vi "Next floor logic. 2vi.vi"(9 "Elevator states array":T1[](array[typedef]), 11 "Floors to serve":cluster{"H call":dbl, "Up":bool}[](array[cluster])) -> (1 "Elevator states array out":T1[](array[typedef]), 3 "Floors to serve out":cluster{"H call":dbl, "Up":bool}[](array[cluster]))   [LabVIEW 2019]
uses:
  Type defs/Elevator states.ctl
  Type defs/Elevator position.ctl
  Type defs/Car buttons.ctl
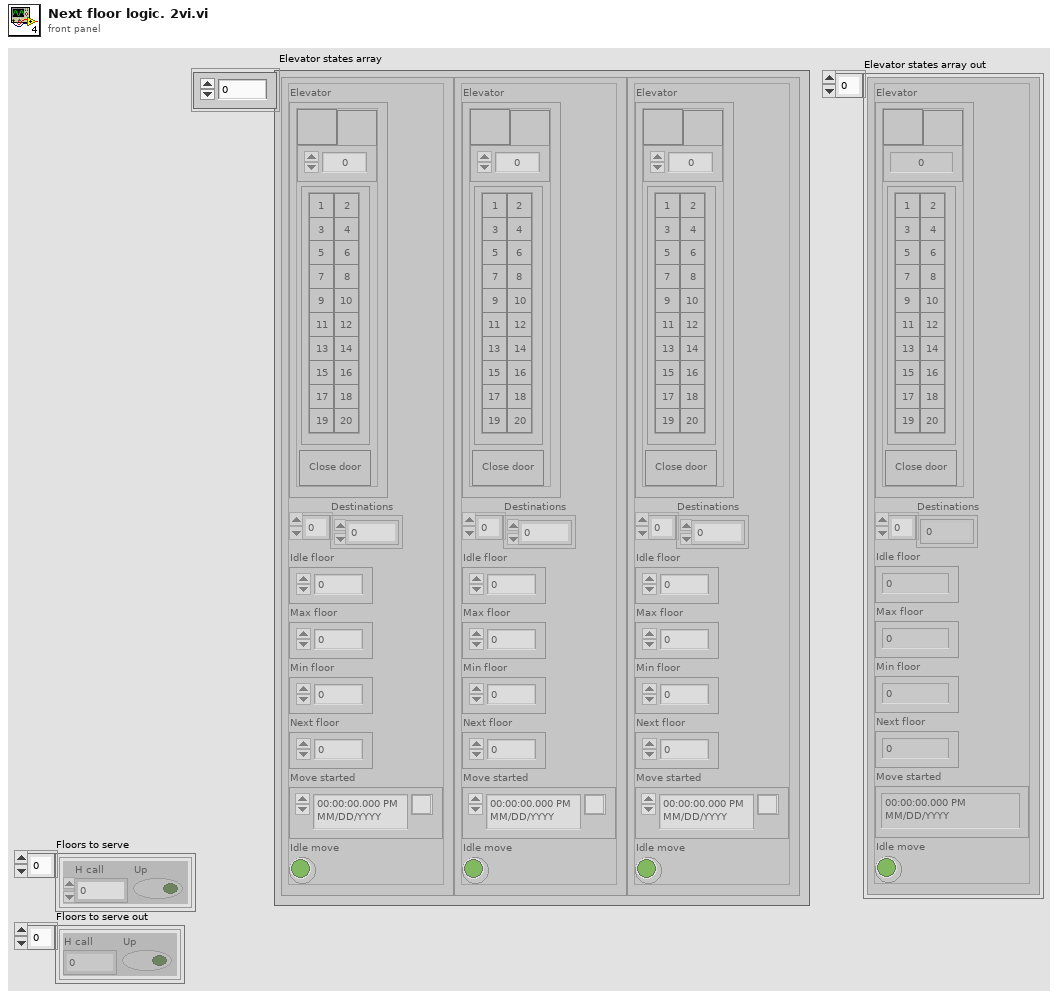
[diagram p1: front panel]
types:
  T1 = typedef "Elevator states.ctl" = cluster{"Elevator":T2, "Destinations":i32[], "Idle floor":u16, "Max floor":u16, "Min floor":u16, "Next floor":u16, "Move started":timestamp, "Idle move":bool}
  T2 = typedef "Elevator position.ctl" = cluster{"Up Button":bool, "Current floor":u16, "Down Button":bool, "Car":T3, "Close door":bool}
  T3 = typedef "Car buttons.ctl" = cluster{"Blank Button":bool, "Blank Button 2":bool, "Blank Button 3":bool, "Blank Button 4":bool, "Blank Button 5":bool, "Blank Button 6":bool, "Blank Button 7":bool, "Blank Button 8":bool, "Blank Button 9":bool, "Blank Button 10":bool, "Blank Button 11":bool, "Blank Button 12":bool, "Blank Button 13":bool, "Blank Button 14":bool, "Blank Button 15":bool, "Blank Button 16":bool, "Blank Button 17":bool, "Blank Button 18":bool, "Blank Button 19":bool, "Blank Button 20":bool}
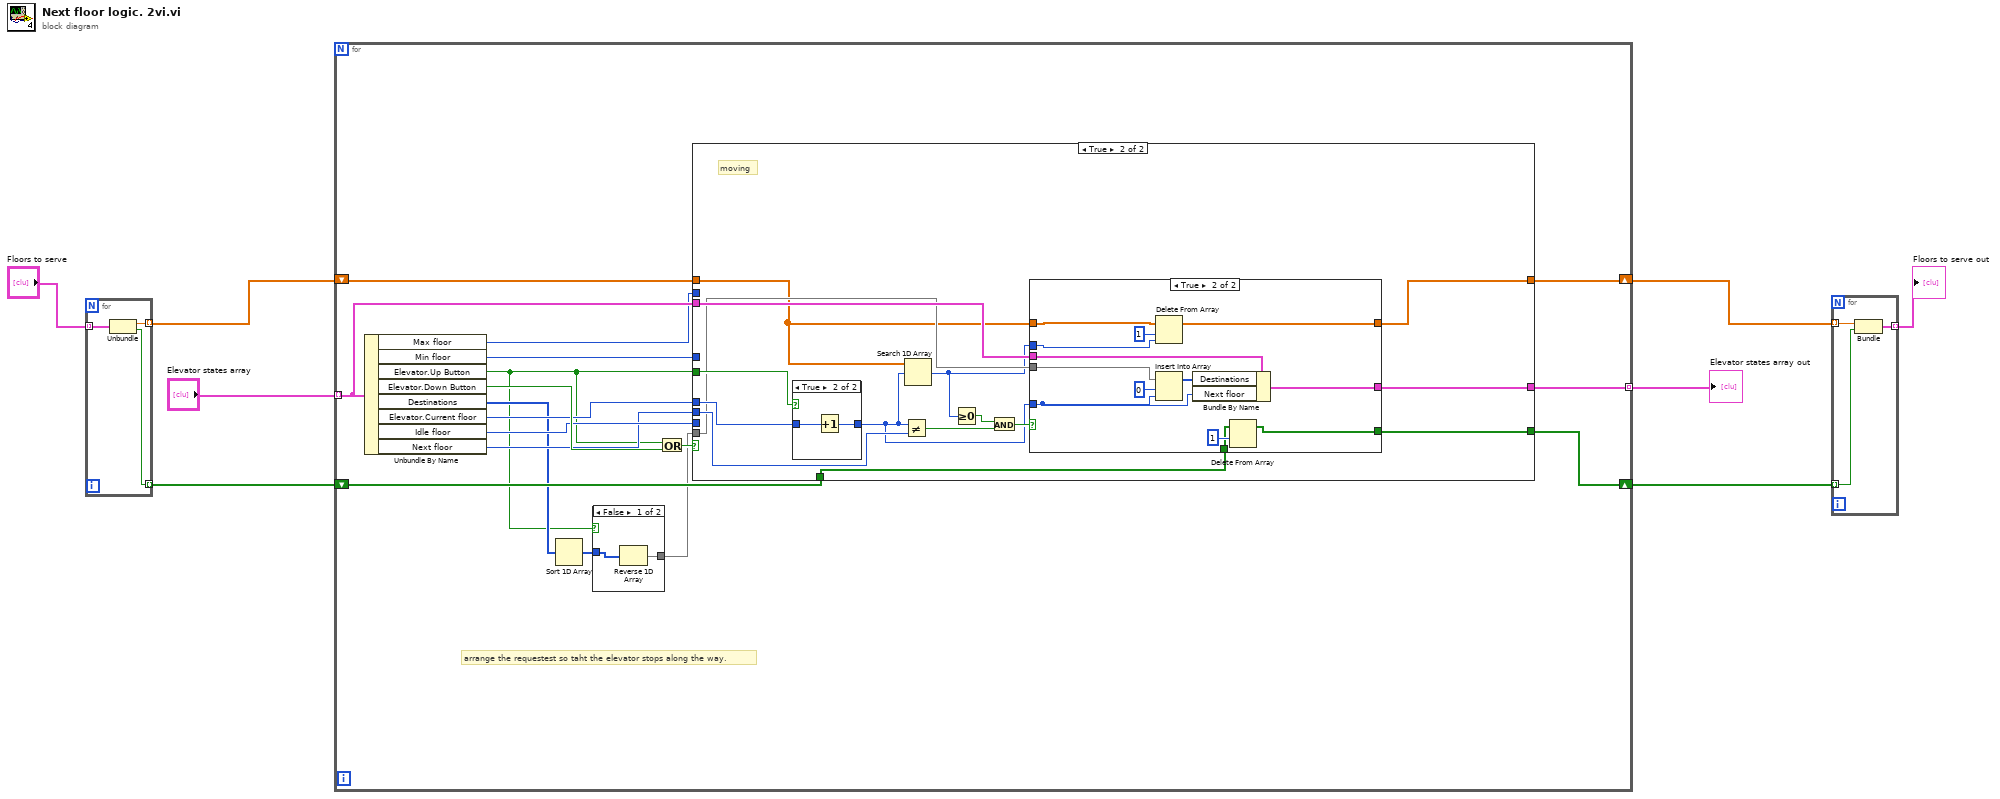
[diagram p0: block diagram]
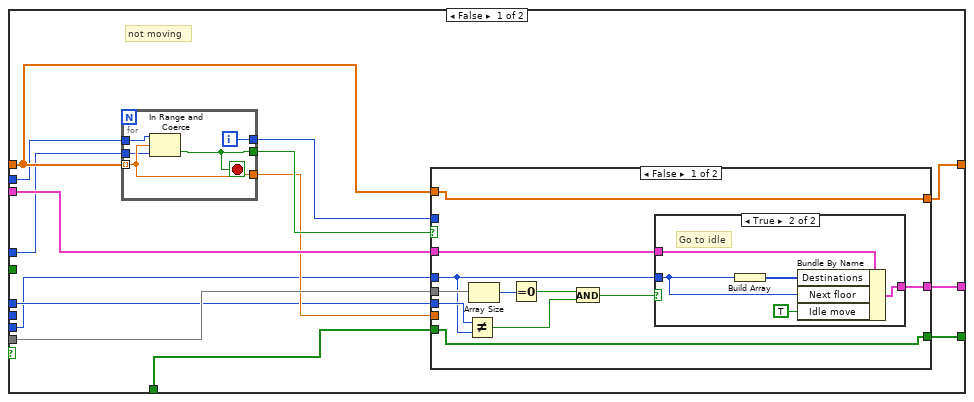
[diagram p3: hidden frame]
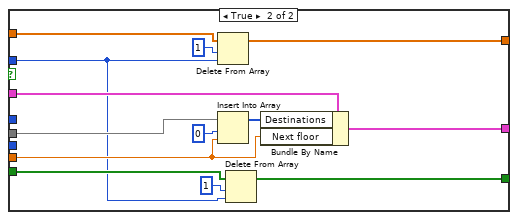
[diagram p5: hidden frame]
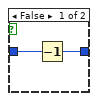
[diagram p7: hidden frame]
diagram:
  n1 = for {
    tunnel: "Floors to serve" -> [w11] mode=indexing
    tunnel: [w10] -> w5 mode=indexing
    tunnel: [w9] -> w2 mode=indexing
    n2 = Unbundle(w11) -> ("H call"=w10:dbl, "Up"=w9:bool)
  }
  n3 = for {
    tunnel: "Elevator states array" -> [w25] mode=indexing
    shift-right: [w24] -> w4
    shift-left: w5 -> [w26]
    tunnel: [w23] -> w7 mode=indexing
    shift-right: [w16] -> w1
    shift-left: w2 -> [w17]
    # "arrange the requestest so taht the elevator stops along the way."
    n4 = Unbundle By Name(w25) -> ("Max floor"=w22:u16, "Min floor"=w21:u16, "Elevator.Up Button"=w14:bool, "Elevator.Down Button"=w28:bool, "Destinations"=w15:i32[], "Elevator.Current floor"=w20:u16, "Idle floor"=w19:u16, "Next floor"=w18:u16)
    n5 = Sort 1D Array(array=w15) -> (sorted array=w12:i32[])
    n6 = case shown="False" w14 {
      tunnel: [w30 w31] -> w13
      tunnel: w12 -> [w29 w31]
      frame False {
        n7 = Reverse 1D Array(array=w29) -> (reversed array=w30:i32[])
      }
      frame True {
      }
    }
    n8 = Or(x=w14, y=w28) -> (x .or. y?=w27:bool)
    n9 = case shown="True" w27 {
      tunnel: w26 -> [w40 w87]
      tunnel: w25 -> [w44 w92]
      tunnel: w13 -> [w43 w88]
      tunnel: [w38 w85] -> w24
      tunnel: [w41 w83] -> w23
      tunnel: w22 -> [w37 _]
      tunnel: w21 -> [w36 _]
      tunnel: w20 -> [w35 w94]
      tunnel: w19 -> [w34 _]
      tunnel: w14 -> [_ w95]
      tunnel: w18 -> [_ w91]
      tunnel: w17 -> [w33 w82]
      tunnel: [w32 w81] -> w16
      frame False {
        # "not moving"
        n10 = for {
          tunnel: w40 -> [w50] mode=indexing
          tunnel: [w46] -> w45
          tunnel: [w50] -> w42
          tunnel: [w49] -> w39
          tunnel: w37 -> [w48]
          tunnel: w36 -> [w47]
          i -> [w49]
          stop <- w46 stop-if-true
          n11 = In Range and Coerce(upper limit=w48, x=w50, lower limit=w47) -> (In Range?=w46:bool)  [unwired: 1 out]
        }
        n12 = case shown="False" w45 {
          tunnel: w44 -> [w54 w80]
          tunnel: w43 -> [w60 w79]
          tunnel: w42 -> [_ w73]
          tunnel: [w53 w77] -> w41
          tunnel: w40 -> [w61 w75]
          tunnel: w39 -> [_ w68]
          tunnel: [w61 w74] -> w38
          tunnel: w35 -> [w58 _]
          tunnel: w34 -> [w52 _]
          tunnel: w33 -> [w51 w70]
          tunnel: [w51 w69] -> w32
          frame False {
            n13 = Not Equal?(x=w58, y=w52) -> (x != y?=w56:bool)
            n14 = Array Size(array=w60) -> (size(s)=w59:i32)
            n15 = Equal To 0?(x=w59) -> (x = 0?=w57:bool)
            n16 = And(x=w57, y=w56) -> (x .and. y?=w55:bool)
            n17 = case shown="True" w55 {
              tunnel: w54 -> [w62 w67]
              tunnel: [w62 w66] -> w53
              tunnel: w52 -> [_ w64]
              frame False {
                # "Already at idle"
              }
              frame True {
                # "Go to idle"
                n18 = Build Array(w64) -> (w65:u16[])
                n19 = Bundle By Name(cluster=w67, "Destinations"=w65, "Next floor"=w64, "Idle move"=TRUE) -> (w66:T1)
              }
            }
          }
          frame True {
            n20 = Delete From Array(array=w75, length=1, index=w68) -> (array with subset deleted=w74:dbl[])  [unwired: 1 out]
            n21 = Insert Into Array(array=w79, index=0, new element=w73) -> (w78:i32[])
            n22 = Delete From Array(array=w70, length=1, index=w68) -> (array with subset deleted=w69:bool[])  [unwired: 1 out]
            n23 = Bundle By Name(cluster=w80, "Destinations"=w78, "Next floor"=w73) -> (w77:T1)
          }
        }
      }
      frame True {
        # "moving"
        n24 = case shown="True" w95 {
          tunnel: w94 -> [w113 w115]
          tunnel: [w112 w114] -> w84
          frame False {
            n25 = Decrement(x=w113) -> (x-1=w112:u16)
          }
          frame True {
            n26 = Increment(x=w115) -> (x+1=w114:u16)
          }
        }
        n27 = Not Equal?(x=w84, y=w91) -> (x != y?=w89:bool)
        n28 = Search 1D Array(1D array=w87, element=w84) -> (index of element=w86:i32)  [unwired: 1 in]
        n29 = Greater Or Equal To 0?(x=w86) -> (x >= 0?=w93:bool)
        n30 = And(x=w93, y=w89) -> (x .and. y?=w90:bool)
        n31 = case shown="True" w90 {
          tunnel: w92 -> [w98 w111]
          tunnel: w88 -> [_ w110]
          tunnel: w87 -> [w97 w107]
          tunnel: w86 -> [_ w106]
          tunnel: [w97 w104] -> w85
          tunnel: w84 -> [_ w103]
          tunnel: [w98 w102] -> w83
          tunnel: w82 -> [w96 w100]
          tunnel: [w96 w99] -> w81
          frame False {
          }
          frame True {
            n32 = Delete From Array(array=w107, length=1, index=w106) -> (array with subset deleted=w104:dbl[])  [unwired: 1 out]
            n33 = Insert Into Array(array=w110, index=0, new element=w103) -> (w108:i32[])
            n34 = Bundle By Name(cluster=w111, "Destinations"=w108, "Next floor"=w103) -> (w102:T1)
            n35 = Delete From Array(array=w100, length=1) -> (array with subset deleted=w99:bool[])  [unwired: 1 in, 1 out]
          }
        }
      }
    }
  }
  "Elevator states array out" <- w7
  n36 = for {
    tunnel: w4 -> [w118] mode=indexing
    tunnel: [w117] -> w3 mode=indexing
    tunnel: w1 -> [w116] mode=indexing
    n37 = Bundle("H call"=w118, "Up"=w116) -> (w117:cluster{"H call":dbl, "Up":bool})  [unwired: 1 in]
  }
  "Floors to serve out" <- w3
